vi "Vol-Path manager.vi"(11 "error in (no error)":errorcluster) -> (4 "File path OK":bool, 6 "Valid data type (& valid path)":bool, 8 "Functional data type":T1, 10 "Speed Data folder path+dummy filename":path, 15 "error":errorcluster)   [LabVIEW 2017]
uses:
  Typedefs/Functional data family.ctl
  Timelapse Viewer/Globals/gl_Time series viewer globals.vi
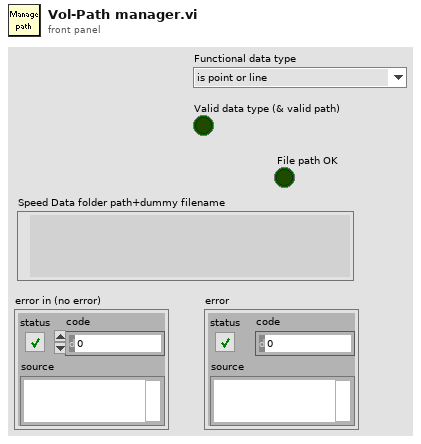
[diagram p1: front panel]
types:
  T1 = typedef "Functional data family.ctl" = enum16{"is point or line", "is surface or volume"}
  T2 = typedef "Time series viewer refs.ctl" = cluster{"This VI":refnum<vi>, "Image control":refnum<vi>, "AVI Mode ind":refnum<vi>, "Play":refnum<vi>, "Stop":refnum<vi>, "Back":refnum<vi>, "Scrollbar":refnum<vi>, "Video length info":refnum<vi>, "Expected speed values":refnum<vi>, "Intensity":refnum<vi>, "Path":refnum<vi>, "Selection sliders":refnum<vi>, "Speed Graph ref":refnum<vi>, "Frame rate set (fps)":refnum<vi>, "Channel to load":refnum<vi>, "Number of rows to generate":refnum<vi>, "Colour":refnum<vi>}
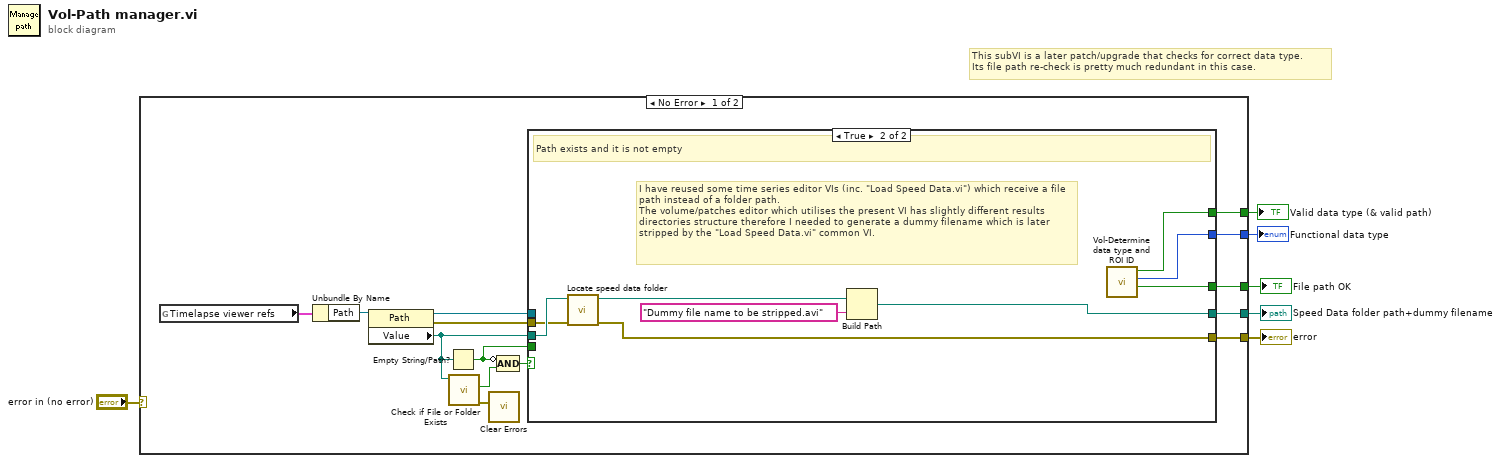
[diagram p0: block diagram]
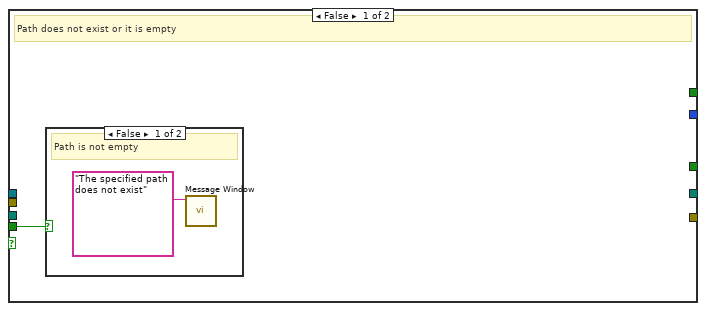
[diagram p2: hidden frame]
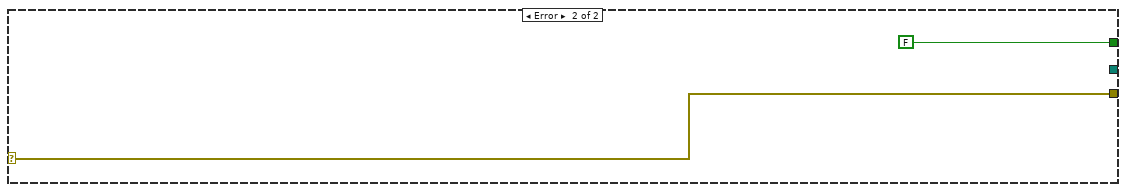
[diagram p4: hidden frame]
diagram:
  # "This subVI is a later patch/upgrade that checks for correct data type.\nIts file path re-check is pretty much redundant in this case."
  n1 = case shown="No Error" "error in (no error)" {
    selector: "error in (no error)" -> [_ w32]
    tunnel: [w18 FALSE ("File path OK 2")] -> w6
    tunnel: [w16 _] -> w5
    tunnel: [w14 w32] -> w3
    tunnel: [w8 _] -> w1
    tunnel: [w7 _] -> w2
    frame No Error {
      n2 = global read "gl_Time series viewer globals.vi" "Timelapse viewer refs"() -> (w19:T2)
      n3 = Unbundle By Name(w19) -> ("Path"=w20:refnum<vi>)
      n4 = property class="Path"(reference=w20) -> (reference out=w17:refnum<vi>, error out=w15:errorcluster, "Value"=w12:path)  [unwired: 1 in]
      n5 = Empty String/Path?(string/path=w12) -> (empty?=w9:bool)
      n6 = call <vilib>:"Check if File or Folder Exists.vi"("path"=w12) -> ("error out"=w13:errorcluster, "file or folder exists?"=w11:bool)  [unwired: 8 in, 1 out]
      n7 = call <vilib>:"Clear Errors.vi"("error in (no error)"=w13) -> ()  [unwired: 5 in, 2 out]
      n8 = Compound Arithmetic op=AND(invert w9, w11) -> (w10:bool)
      n9 = case shown="True" w10 {
        tunnel: [_ w25] -> w18
        tunnel: w17 -> [_ _]
        tunnel: [_ w26] -> w16
        tunnel: w15 -> [_ w30]
        tunnel: [_ w29] -> w14
        tunnel: w12 -> [_ w31]
        tunnel: w9 -> [w21 _]
        tunnel: [_ w24] -> w8
        tunnel: [_ w23] -> w7
        frame False {
          # "Path does not exist or it is empty"
          n10 = case shown="False" w21 {
            frame False {
              # "Path is not empty"
              n11 = call "Message Window.vi"("Message string"="The specified path does not exist") -> ()  [unwired: 10 in, 1 out]
            }
            frame True {
              # "Path is empty"
            }
          }
        }
        frame True {
          # "I have reused some time series editor VIs (inc. \"Load Speed Data.vi\") which receive a file path instead of a folder path.\nThe volume/patches editor which utilises the present VI has slightly different results directories structure therefore I needed to generate a dummy filename which is later stripped by the \"Load Speed Data.vi\" common VI."
          # "Path exists and it is not empty"
          n12 = call "Locate speed data folder.vi"("error in (no error)"=w30, "Value"=w31) -> ("error out"=w29:errorcluster, "Speed data folder's path"=w28:path)  [unwired: 8 in]
          n13 = Build Path(base path=w28, name or relative path="Dummy file name to be stripped.avi") -> (appended path=w26:path)
          n14 = call "Vol-Determine data type and ROI ID.vi"() -> ("Valid path"=w25:bool, "Functional data type"=w24:T1, "Valid data type"=w23:bool)  [unwired: 8 in, 1 out]
        }
      }
    }
    frame Error {
    }
  }
  "File path OK" <- w6
  "Speed Data folder path+dummy filename" <- w5
  "error" <- w3
  "Valid data type (& valid path)" <- w2
  "Functional data type" <- w1
